vi "ArmXZConstants.vi"() -> (1 "Unextended Length (in)":dbl, 3 "Pivot Height (in)":dbl)   [LabVIEW 2020]
doc: "Constants for XYZ\nOutputs:\n--Pivot Height--Double--Inches\n--Unextended Length--Double"
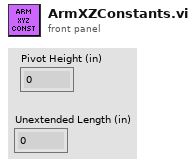
[diagram p1: front panel]
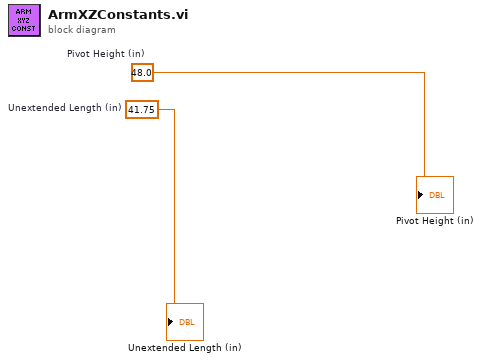
[diagram p0: block diagram]
diagram:
  w2 = 48.0  # Pivot Height (in)
  w1 = 41.75  # Unextended Length (in)
  "Pivot Height (in)" <- w2
  "Unextended Length (in)" <- w1
